vi "Terminal-Main-SelfCheck.vi"() -> ()   [LabVIEW 2014]
panel:
  out "簇":T1
  out "传感器数据采集":bool
  out "动力子系统":bool
  out "齿轮子系统":bool
  out "液压子系统":bool
  in  "最大尝试次数（5）":i32=5
  out "error out":errorcluster caption="错误输出"
  in  "error in (no error)":errorcluster caption="错误输入（无错误）"
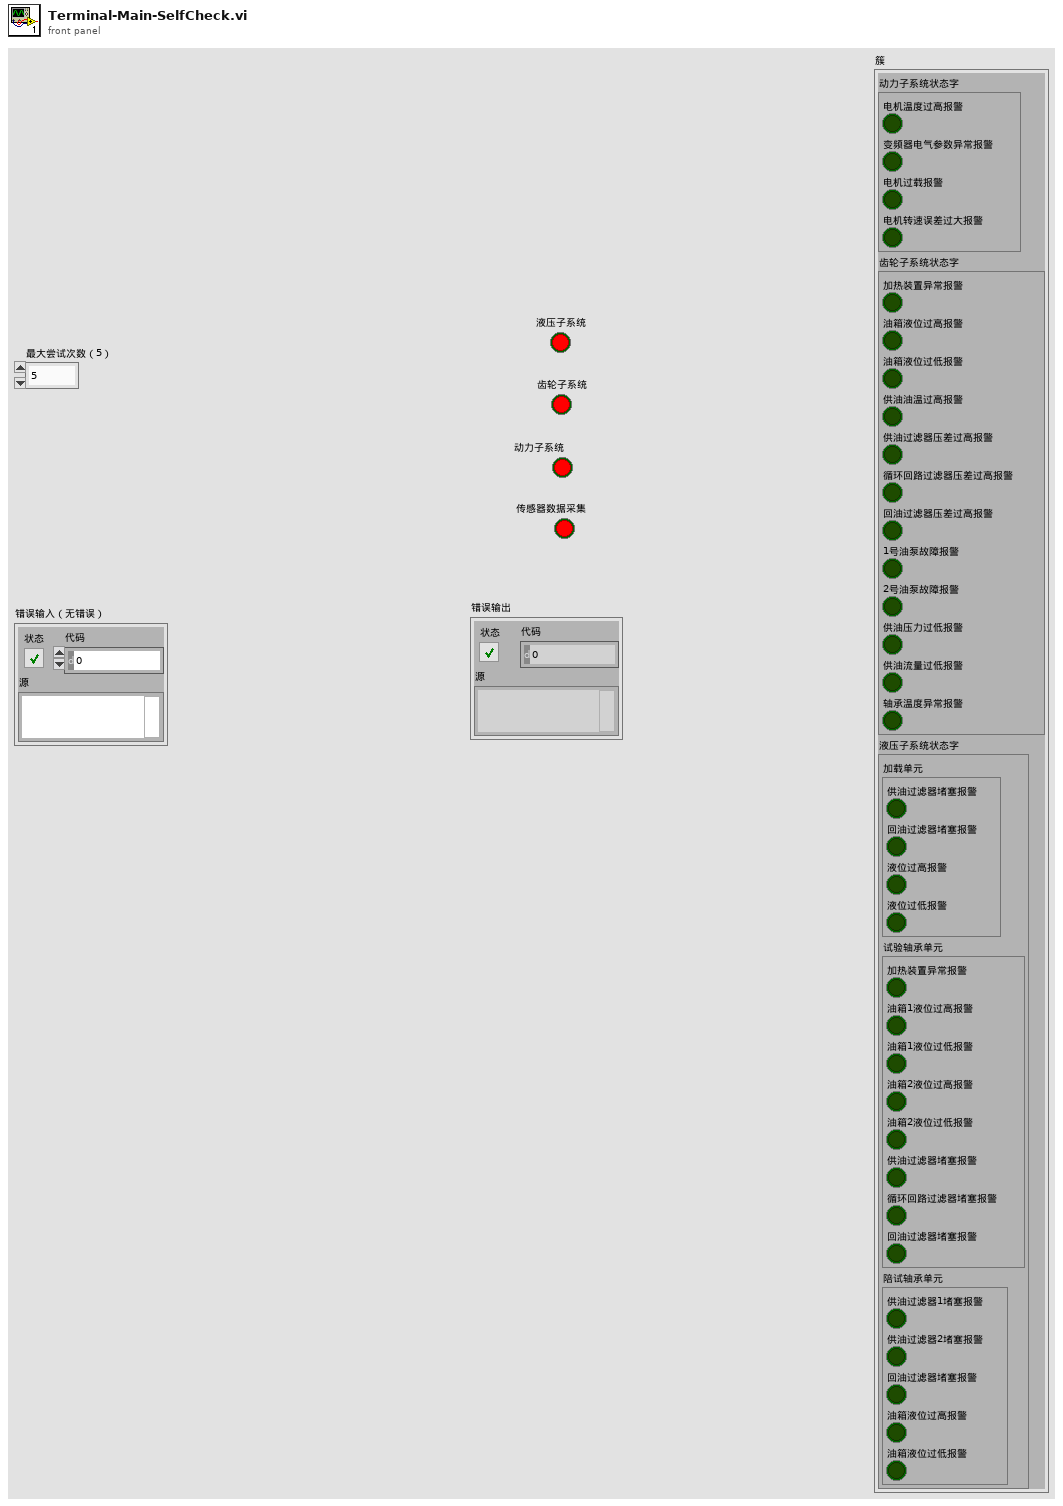
[diagram p1: front panel]
types:
  T1 = cluster{"动力子系统状态字":cluster{"电机温度过高报警":bool, "变频器电气参数异常报警":bool, "电机过载报警":bool, "电机转速误差过大报警":bool}, "齿轮子系统状态字":cluster{"加热装置异常报警":bool, "油箱液位过高报警":bool, "油箱液位过低报警":bool, "供油油温过高报警":bool, "供油过滤器压差过高报警":bool, "循环回路过滤器压差过高报警":bool, "回油过滤器压差过高报警":bool, "1号油泵故障报警":bool, "2号油泵故障报警":bool, "供油压力过低报警":bool, "供油流量过低报警":bool, "轴承温度异常报警":bool}, "液压子系统状态字":cluster{"加载单元":cluster{"供油过滤器堵塞报警":bool, "回油过滤器堵塞报警":bool, "液位过高报警":bool, "液位过低报警":bool}, "试验轴承单元":cluster{"加热装置异常报警":bool, "油箱1液位过高报警":bool, "油箱1液位过低报警":bool, "油箱2液位过高报警":bool, "油箱2液位过低报警":bool, "供油过滤器堵塞报警":bool, "循环回路过滤器堵塞报警":bool, "回油过滤器堵塞报警":bool}, "陪试轴承单元":cluster{"供油过滤器1堵塞报警":bool, "供油过滤器2堵塞报警":bool, "回油过滤器堵塞报警":bool, "油箱液位过高报警":bool, "油箱液位过低报警":bool}}}
  T2 = cluster{"加载单元":cluster{"供油过滤器堵塞报警":bool, "回油过滤器堵塞报警":bool, "液位过高报警":bool, "液位过低报警":bool}, "试验轴承单元":cluster{"加热装置异常报警":bool, "油箱1液位过高报警":bool, "油箱1液位过低报警":bool, "油箱2液位过高报警":bool, "油箱2液位过低报警":bool, "供油过滤器堵塞报警":bool, "循环回路过滤器堵塞报警":bool, "回油过滤器堵塞报警":bool}, "陪试轴承单元":cluster{"供油过滤器1堵塞报警":bool, "供油过滤器2堵塞报警":bool, "回油过滤器堵塞报警":bool, "油箱液位过高报警":bool, "油箱液位过低报警":bool}}
  T3 = cluster{"加热装置异常报警":bool, "油箱液位过高报警":bool, "油箱液位过低报警":bool, "供油油温过高报警":bool, "供油过滤器压差过高报警":bool, "循环回路过滤器压差过高报警":bool, "回油过滤器压差过高报警":bool, "1号油泵故障报警":bool, "2号油泵故障报警":bool, "供油压力过低报警":bool, "供油流量过低报警":bool, "轴承温度异常报警":bool}
  T4 = cluster{"变送器配电模块电压":u16, "变频器电流":u16, "变频器电压":u16, "变频器频率":u16, "动力子系统状态字":cluster{"电机温度过高报警":bool, "变频器电气参数异常报警":bool, "电机过载报警":bool, "电机转速误差过大报警":bool}}
  T5 = cluster{"电机温度过高报警":bool, "变频器电气参数异常报警":bool, "电机过载报警":bool, "电机转速误差过大报警":bool}
  T6 = cluster{"润滑油流量":u16, "油箱润滑油液位":u16, "油箱温度":u16, "供油压力":u16, "过滤器压差":u16, "油箱液位":u16, "供油油温":u16, "齿轮箱轴承温度":u16, "齿轮箱高速端输出转速":u16, "齿轮子系统状态字":cluster{"加热装置异常报警":bool, "油箱液位过高报警":bool, "油箱液位过低报警":bool, "供油油温过高报警":bool, "供油过滤器压差过高报警":bool, "循环回路过滤器压差过高报警":bool, "回油过滤器压差过高报警":bool, "1号油泵故障报警":bool, "2号油泵故障报警":bool, "供油压力过低报警":bool, "供油流量过低报警":bool, "轴承温度异常报警":bool}}
  T7 = cluster{"径向油缸加载压力":u16, "轴向油缸加载压力":u16, "油箱1油液温度":u16, "润滑油温度":u16, "油箱2油液温度":u16, "试验轴承供油压力":u16, "试验轴承供油流量":u16, "陪试轴承供油流量":u16, "陪试轴承供油压力":u16, "陪试轴承供油温度":u16, "液压子系统状态字":cluster{"加载单元":cluster{"供油过滤器堵塞报警":bool, "回油过滤器堵塞报警":bool, "液位过高报警":bool, "液位过低报警":bool}, "试验轴承单元":cluster{"加热装置异常报警":bool, "油箱1液位过高报警":bool, "油箱1液位过低报警":bool, "油箱2液位过高报警":bool, "油箱2液位过低报警":bool, "供油过滤器堵塞报警":bool, "循环回路过滤器堵塞报警":bool, "回油过滤器堵塞报警":bool}, "陪试轴承单元":cluster{"供油过滤器1堵塞报警":bool, "供油过滤器2堵塞报警":bool, "回油过滤器堵塞报警":bool, "油箱液位过高报警":bool, "油箱液位过低报警":bool}}}
  T8 = cluster{"供油过滤器堵塞报警":bool, "回油过滤器堵塞报警":bool, "液位过高报警":bool, "液位过低报警":bool}
  T9 = cluster{"加热装置异常报警":bool, "油箱1液位过高报警":bool, "油箱1液位过低报警":bool, "油箱2液位过高报警":bool, "油箱2液位过低报警":bool, "供油过滤器堵塞报警":bool, "循环回路过滤器堵塞报警":bool, "回油过滤器堵塞报警":bool}
  T10 = cluster{"供油过滤器1堵塞报警":bool, "供油过滤器2堵塞报警":bool, "回油过滤器堵塞报警":bool, "油箱液位过高报警":bool, "油箱液位过低报警":bool}
  T11 = cluster{"时间":timestamp, "声发射":sgl[], "电涡流1":sgl[], "电涡流2":sgl[], "电涡流3":sgl[], "电涡流4":sgl[], "电涡流5":sgl[], "加速度1":sgl[], "加速度2":sgl[]}
  T12 = cluster{"时间":timestamp, "陪试轴承润滑单元出油温度1":sgl[], "陪试轴承润滑单元出油温度2":sgl[], "轴承外圈温度":sgl[], "出油温度":sgl[], "摩擦力1":sgl[], "摩擦力2":sgl[], "径向油缸力":sgl[], "轴向油缸力":sgl[], "转速":sgl[]}
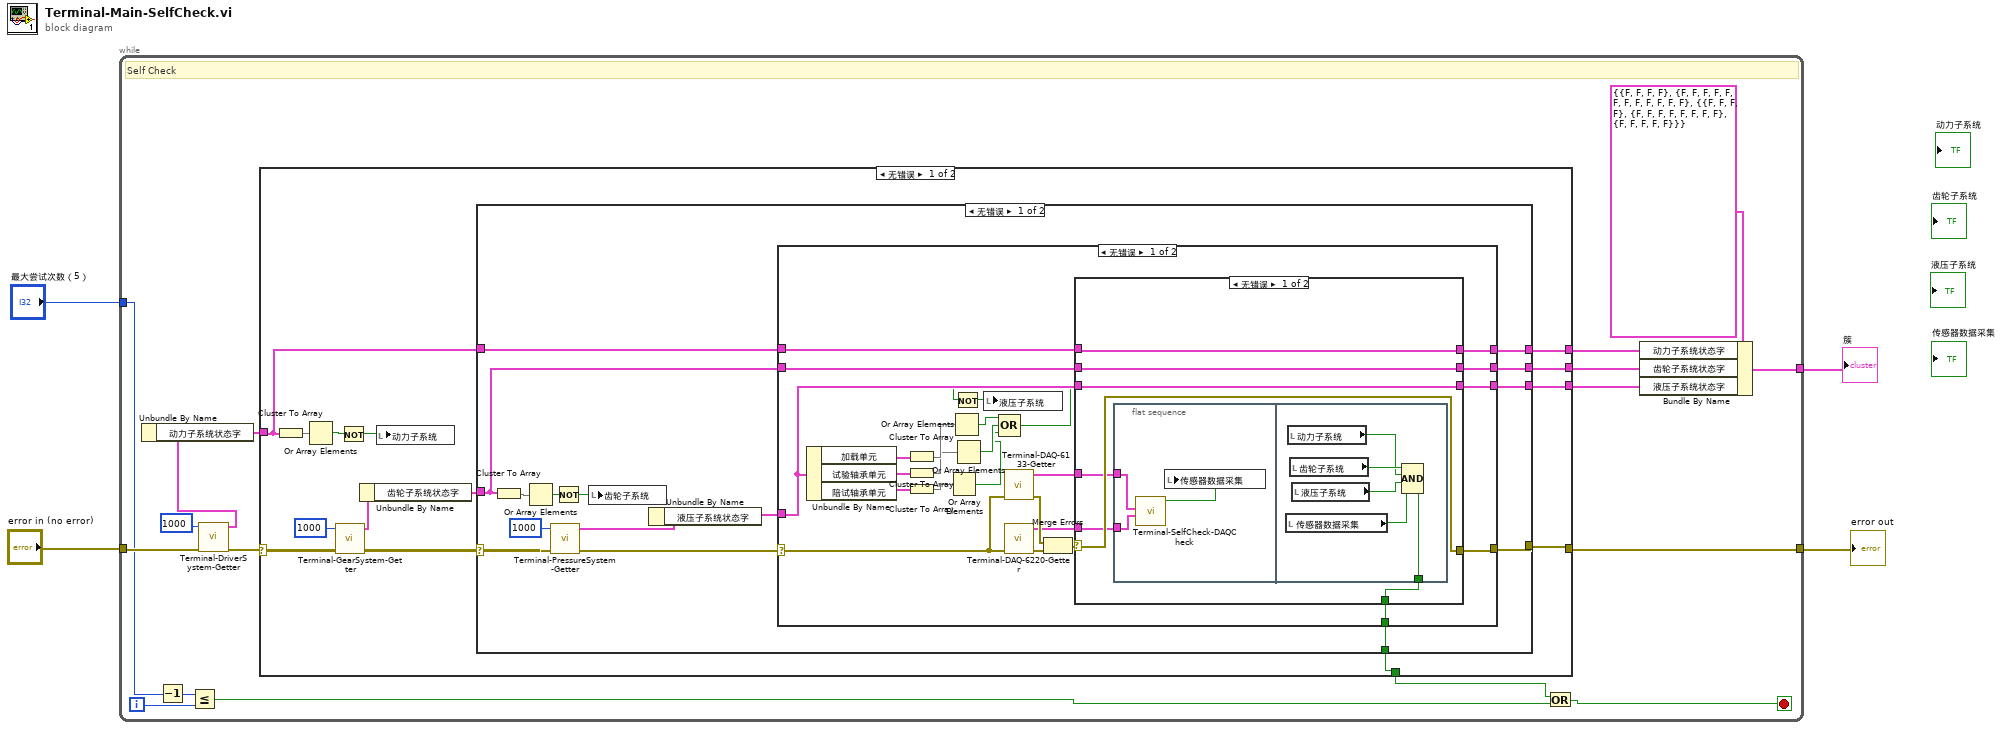
[diagram p0: block diagram]
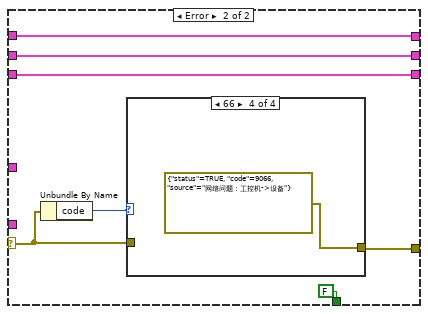
[diagram p2: hidden frame]
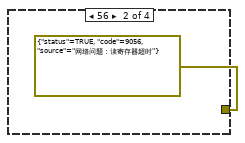
[diagram p4: hidden frame]
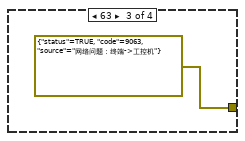
[diagram p5: hidden frame]
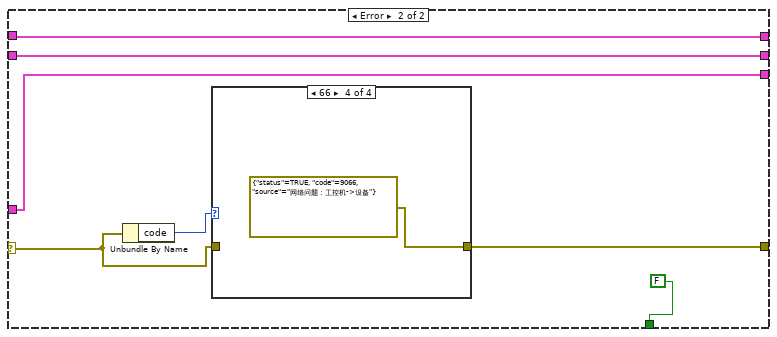
[diagram p6: hidden frame]
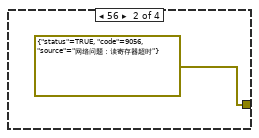
[diagram p8: hidden frame]
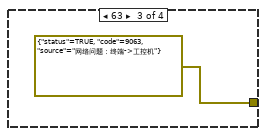
[diagram p9: hidden frame]
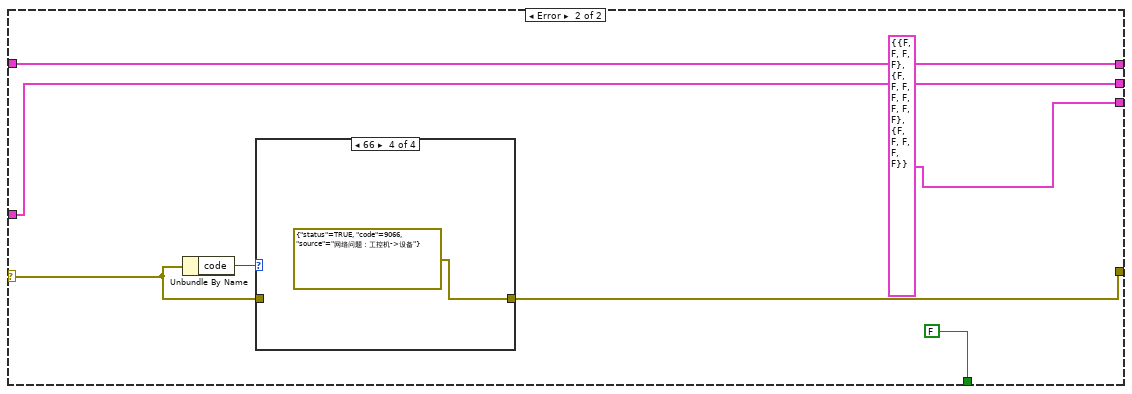
[diagram p10: hidden frame]
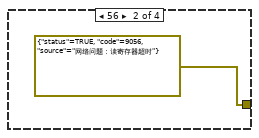
[diagram p12: hidden frame]
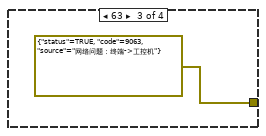
[diagram p13: hidden frame]
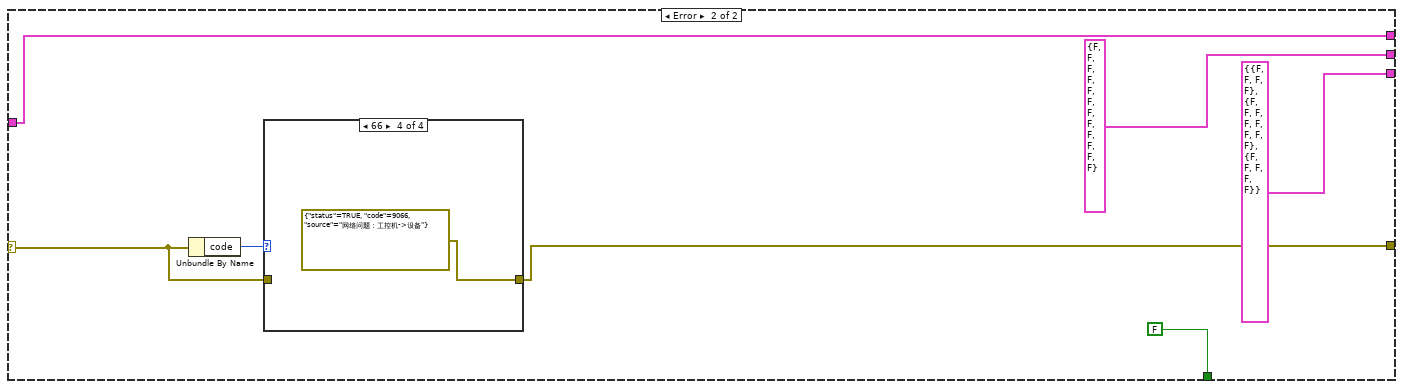
[diagram p14: hidden frame]
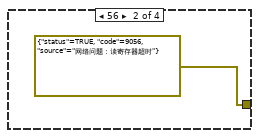
[diagram p16: hidden frame]
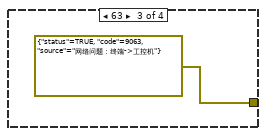
[diagram p17: hidden frame]
diagram:
  n1 = while {
    tunnel: "最大尝试次数（5）" -> [w8]
    tunnel: [w12] -> w1
    tunnel: "error in (no error)" -> [w21]
    tunnel: [w11] -> w3
    i -> [w10]
    stop <- w16 stop-if-true
    # "Self Check"
    n2 = Decrement(x=w8) -> (x-1=w9:i32)
    n3 = Less Or Equal?(x=w9, y=w10) -> (x <= y?=w15:bool)
    n4 = call "Terminal-DriverSystem-Getter.vi"("error in (no error)"=w21, "read operation timeout (ms)"=1000) -> ("error out"=w19:errorcluster, "设备信息"=w18:T4)  [unwired: 7 in, 1 out]
    n5 = Unbundle By Name(w18) -> ("动力子系统状态字"=w17:T5)
    n6 = case shown="无错误" w19 {
      selector: w19 -> [w34 w127]
      tunnel: w17 -> [w27 w129]
      tunnel: [w26 FALSE] -> w14
      tunnel: [w25 w129] -> w13
      tunnel: [w24 T3 {"加热装置异常报警"=FALSE, "油箱液位过高报警"=FALSE, "油箱液位过低报警"=FALSE, "供油油温过高报警"=FALSE, "供油过滤器压差过高报警"=FALSE, "循环回路过滤器压差过高报警"=FALSE, "回油过滤器压差过高报警"=FALSE, "1号油泵故障报警"=FALSE, "2号油泵故障报警"=FALSE, "供油压力过低报警"=FALSE, "供油流量过低报警"=FALSE, "轴承温度异常报警"=FALSE} ("齿轮子系统状态字")] -> w7
      tunnel: [w22 T2 {"加载单元"={"供油过滤器堵塞报警"=FALSE, "回油过滤器堵塞报警"=FALSE, "液位过高报警"=FALSE, "液位过低报警"=FALSE}, "试验轴承单元"={"加热装置异常报警"=FALSE, "油箱1液位过高报警"=FALSE, "油箱1液位过低报警"=FALSE, "油箱2液位过高报警"=FALSE, "油箱2液位过低报警"=FALSE, "供油过滤器堵塞报警"=FALSE, "循环回路过滤器堵塞报警"=FALSE, "回油过滤器堵塞报警"=FALSE}, "陪试轴承单元"={"供油过滤器1堵塞报警"=FALSE, "供油过滤器2堵塞报警"=FALSE, "回油过滤器堵塞报警"=FALSE, "油箱液位过高报警"=FALSE, "油箱液位过低报警"=FALSE}} ("液压子系统状态字")] -> w5
      tunnel: [w23 w126] -> w11
      frame No Error {
        n7 = Cluster To Array(cluster=w27) -> (array=w29:bool[])
        n8 = Or Array Elements(Boolean array=w29) -> (logical OR=w28:bool)
        n9 = call "Terminal-GearSystem-Getter.vi"("error in (no error)"=w34, "read operation timeout (ms)"=1000) -> ("error out"=w32:errorcluster, "设备信息"=w31:T6)  [unwired: 7 in, 1 out]
        n10 = Not(x=w28) -> (.not. x?=w35:bool)
        n11 = Unbundle By Name(w31) -> ("齿轮子系统状态字"=w30:T3)
        n12 = local write "动力子系统"(w35) -> ()
        n13 = case shown="无错误" w32 {
          selector: w32 -> [w47 w115]
          tunnel: w30 -> [w42 w118]
          tunnel: w27 -> [w43 w117]
          tunnel: [w41 FALSE] -> w26
          tunnel: [w40 w117] -> w25
          tunnel: [w39 w118] -> w24
          tunnel: [w36 T2 {"加载单元"={"供油过滤器堵塞报警"=FALSE, "回油过滤器堵塞报警"=FALSE, "液位过高报警"=FALSE, "液位过低报警"=FALSE}, "试验轴承单元"={"加热装置异常报警"=FALSE, "油箱1液位过高报警"=FALSE, "油箱1液位过低报警"=FALSE, "油箱2液位过高报警"=FALSE, "油箱2液位过低报警"=FALSE, "供油过滤器堵塞报警"=FALSE, "循环回路过滤器堵塞报警"=FALSE, "回油过滤器堵塞报警"=FALSE}, "陪试轴承单元"={"供油过滤器1堵塞报警"=FALSE, "供油过滤器2堵塞报警"=FALSE, "回油过滤器堵塞报警"=FALSE, "油箱液位过高报警"=FALSE, "油箱液位过低报警"=FALSE}} ("液压子系统状态字")] -> w22
          tunnel: [w38 w116] -> w23
          frame No Error {
            n14 = Cluster To Array(cluster=w42) -> (array=w50:bool[])
            n15 = Or Array Elements(Boolean array=w50) -> (logical OR=w49:bool)
            n16 = call "Terminal-PressureSystem-Getter.vi"("error in (no error)"=w47, "read operation timeout (ms)"=1000) -> ("error out"=w46:errorcluster, "设备信息"=w45:T7)  [unwired: 7 in, 1 out]
            n17 = Not(x=w49) -> (.not. x?=w48:bool)
            n18 = local write "齿轮子系统"(w48) -> ()
            n19 = Unbundle By Name(w45) -> ("液压子系统状态字"=w44:T2)
            n20 = case shown="无错误" w46 {
              selector: w46 -> [w67 w102]
              tunnel: w44 -> [w61 w107]
              tunnel: w43 -> [w74 w105]
              tunnel: w42 -> [w73 w106]
              tunnel: [w72 FALSE] -> w41
              tunnel: [w71 w105] -> w40
              tunnel: [w70 w106] -> w39
              tunnel: [w69 w107] -> w36
              tunnel: [w68 w104] -> w38
              frame No Error {
                n21 = Unbundle By Name(w61) -> ("加载单元"=w60:T8, "试验轴承单元"=w59:T9, "陪试轴承单元"=w58:T10)
                n22 = Cluster To Array(cluster=w60) -> (array=w57:bool[])
                n23 = Cluster To Array(cluster=w59) -> (array=w56:bool[])
                n24 = Cluster To Array(cluster=w58) -> (array=w55:bool[])
                n25 = Or Array Elements(Boolean array=w55) -> (logical OR=w52:bool)
                n26 = Or Array Elements(Boolean array=w57) -> (logical OR=w54:bool)
                n27 = Or Array Elements(Boolean array=w56) -> (logical OR=w53:bool)
                n28 = Compound Arithmetic op=OR(w54, w53, w52) -> (w51:bool)
                n29 = Not(x=w51) -> (.not. x?=w75:bool)
                n30 = local write "液压子系统"(w75) -> ()
                n31 = call "Terminal-DAQ-6133-Getter.vi"("error in (no error)"=w67) -> ("error out"=w65:errorcluster, "6133"=w63:T11)  [unwired: 9 in]
                n32 = call "Terminal-DAQ-6220-Getter.vi"("error in (no error)"=w67) -> ("error out"=w66:errorcluster, "6220"=w62:T12)  [unwired: 9 in]
                n33 = Merge Errors(w65, w66) -> (w64:errorcluster)
                n34 = case shown="无错误" w64 {
                  selector: w64 -> [w78 w92]
                  tunnel: w74 -> [w81 w94]
                  tunnel: w73 -> [w80 w95]
                  tunnel: w61 -> [w79 w96]
                  tunnel: [w82 FALSE] -> w72
                  tunnel: [w81 w94] -> w71
                  tunnel: [w80 w95] -> w70
                  tunnel: [w79 w96] -> w69
                  tunnel: [w78 w91] -> w68
                  tunnel: w63 -> [w77 _]
                  tunnel: w62 -> [w76 _]
                  frame No Error {
                    n35 = flat-sequence {
                      tunnel: w77 -> [w84]
                      tunnel: w76 -> [w85]
                      tunnel: [w90] -> w82
                      frame #0 {
                        n36 = call "Terminal-SelfCheck-DAQCheck.vi"("6220"=w85, "6133"=w84) -> ("结果"=w83:bool)  [unwired: 9 in]
                        n37 = local write "传感器数据采集"(w83) -> ()
                      }
                      frame #1 {
                        n38 = local read "传感器数据采集"() -> (w86:bool)
                        n39 = local read "动力子系统"() -> (w89:bool)
                        n40 = local read "齿轮子系统"() -> (w88:bool)
                        n41 = local read "液压子系统"() -> (w87:bool)
                        n42 = Compound Arithmetic op=AND(w89, w88, w87, w86) -> (w90:bool)
                      }
                    }
                  }
                  frame Error {
                    n43 = Unbundle By Name(w92) -> ("code"=w93:i32)
                    n44 = case shown="66" w93 {
                      tunnel: w92 -> [w98 _ _ _]
                      tunnel: [w98 errorcluster {"status"=TRUE, "code"=9056, "source"="网络问题：读寄存器超时"} ("错误常量") errorcluster {"status"=TRUE, "code"=9063, "source"="网络问题：终端->工控机"} ("错误常量") errorcluster {"status"=TRUE, "code"=9066, "source"="网络问题：工控机->设备"} ("错误常量")] -> w91
                      frame Default {
                      }
                      frame 56 {
                      }
                      frame 63 {
                      }
                      frame 66 {
                      }
                    }
                  }
                }
              }
              frame Error {
                n45 = Unbundle By Name(w102) -> ("code"=w103:i32)
                n46 = case shown="66" w103 {
                  tunnel: w102 -> [w109 _ _ _]
                  tunnel: [w109 errorcluster {"status"=TRUE, "code"=9056, "source"="网络问题：读寄存器超时"} ("错误常量") errorcluster {"status"=TRUE, "code"=9063, "source"="网络问题：终端->工控机"} ("错误常量") errorcluster {"status"=TRUE, "code"=9066, "source"="网络问题：工控机->设备"} ("错误常量")] -> w104
                  frame Default {
                  }
                  frame 56 {
                  }
                  frame 63 {
                  }
                  frame 66 {
                  }
                }
              }
            }
          }
          frame Error {
            n47 = Unbundle By Name(w115) -> ("code"=w114:i32)
            n48 = case shown="66" w114 {
              tunnel: w115 -> [w120 _ _ _]
              tunnel: [w120 errorcluster {"status"=TRUE, "code"=9056, "source"="网络问题：读寄存器超时"} ("错误常量") errorcluster {"status"=TRUE, "code"=9063, "source"="网络问题：终端->工控机"} ("错误常量") errorcluster {"status"=TRUE, "code"=9066, "source"="网络问题：工控机->设备"} ("错误常量")] -> w116
              frame Default {
              }
              frame 56 {
              }
              frame 63 {
              }
              frame 66 {
              }
            }
          }
        }
      }
      frame Error {
        n49 = Unbundle By Name(w127) -> ("code"=w128:i32)
        n50 = case shown="66" w128 {
          tunnel: w127 -> [w131 _ _ _]
          tunnel: [w131 errorcluster {"status"=TRUE, "code"=9056, "source"="网络问题：读寄存器超时"} ("错误常量") errorcluster {"status"=TRUE, "code"=9063, "source"="网络问题：终端->工控机"} ("错误常量") errorcluster {"status"=TRUE, "code"=9066, "source"="网络问题：工控机->设备"} ("错误常量")] -> w126
          frame Default {
          }
          frame 56 {
          }
          frame 63 {
          }
          frame 66 {
          }
        }
      }
    }
    n51 = Or(x=w14, y=w15) -> (x .or. y?=w16:bool)
    n52 = Bundle By Name(cluster=T1 {"动力子系统状态字"={"电机温度过高报警"=FALSE, "变频器电气参数异常报警"=FALSE, "电机过载报警"=FALSE, "电机转速误差过大报警"=FALSE}, "齿轮子系统状态字"={"加热装置异常报警"=FALSE, "油箱液位过高报警"=FALSE, "油箱液位过低报警"=FALSE, "供油油温过高报警"=FALSE, "供油过滤器压差过高报警"=FALSE, "循环回路过滤器压差过高报警"=FALSE, "回油过滤器压差过高报警"=FALSE, "1号油泵故障报警"=FALSE, "2号油泵故障报警"=FALSE, "供油压力过低报警"=FALSE, "供油流量过低报警"=FALSE, "轴承温度异常报警"=FALSE}, "液压子系统状态字"={"加载单元"={"供油过滤器堵塞报警"=FALSE, "回油过滤器堵塞报警"=FALSE, "液位过高报警"=FALSE, "液位过低报警"=FALSE}, "试验轴承单元"={"加热装置异常报警"=FALSE, "油箱1液位过高报警"=FALSE, "油箱1液位过低报警"=FALSE, "油箱2液位过高报警"=FALSE, "油箱2液位过低报警"=FALSE, "供油过滤器堵塞报警"=FALSE, "循环回路过滤器堵塞报警"=FALSE, "回油过滤器堵塞报警"=FALSE}, "陪试轴承单元"={"供油过滤器1堵塞报警"=FALSE, "供油过滤器2堵塞报警"=FALSE, "回油过滤器堵塞报警"=FALSE, "油箱液位过高报警"=FALSE, "油箱液位过低报警"=FALSE}}}, "动力子系统状态字"=w13, "齿轮子系统状态字"=w7, "液压子系统状态字"=w5) -> (w12:T1)
  }
  "error out" <- w3
  "簇" <- w1
